vi "ClearAll.vi"(8 "error in":errorcluster) -> (0 "error out":errorcluster)   [LabVIEW 2016]
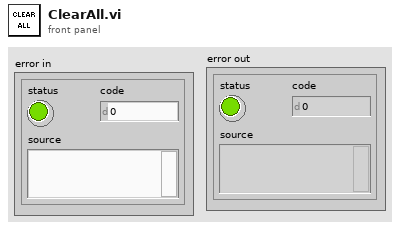
[diagram p1: front panel]
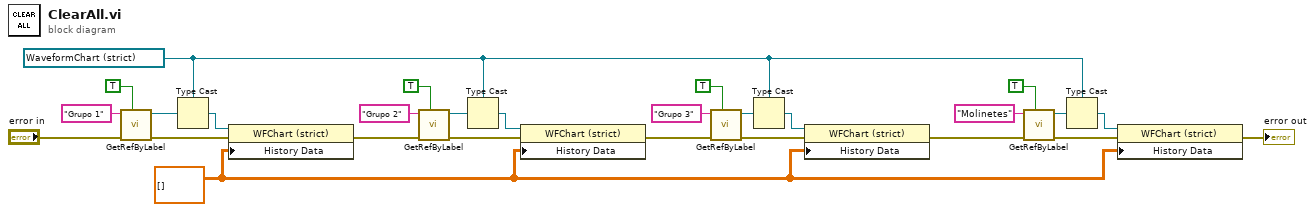
[diagram p0: block diagram]
diagram:
  w4 = dbl[][] [] ("History Data")
  w2 = refnum<vi> refnum ("Grupo 1")
  n1 = call "GetRefByLabel.vi"("InsideTab"=TRUE, "error in"="error in", "Label"="Grupo 1") -> ("error out"=w19:errorcluster, "Ctl Refnum"=w21:refnum<vi>)  [unwired: 6 in, 1 out]
  n2 = Type Cast(type=w2, x=w21) -> (*(type *) &x=w18:refnum<vi>)
  n3 = property class="WFChart (strict)"(reference=w18, error in=w19, "History Data"=w4) -> (error out=w17:errorcluster)  [unwired: 1 out]
  n4 = call "GetRefByLabel.vi"("InsideTab"=TRUE, "error in"=w17, "Label"="Grupo 2") -> ("error out"=w15:errorcluster, "Ctl Refnum"=w16:refnum<vi>)  [unwired: 6 in, 1 out]
  n5 = Type Cast(type=w2, x=w16) -> (*(type *) &x=w14:refnum<vi>)
  n6 = property class="WFChart (strict)"(reference=w14, error in=w15, "History Data"=w4) -> (error out=w13:errorcluster)  [unwired: 1 out]
  n7 = call "GetRefByLabel.vi"("InsideTab"=TRUE, "error in"=w13, "Label"="Grupo 3") -> ("error out"=w11:errorcluster, "Ctl Refnum"=w12:refnum<vi>)  [unwired: 6 in, 1 out]
  n8 = Type Cast(type=w2, x=w12) -> (*(type *) &x=w10:refnum<vi>)
  n9 = property class="WFChart (strict)"(reference=w10, error in=w11, "History Data"=w4) -> (error out=w3:errorcluster)  [unwired: 1 out]
  n10 = call "GetRefByLabel.vi"("InsideTab"=TRUE, "error in"=w3, "Label"="Molinetes") -> ("error out"=w8:errorcluster, "Ctl Refnum"=w7:refnum<vi>)  [unwired: 6 in, 1 out]
  n11 = Type Cast(type=w2, x=w7) -> (*(type *) &x=w9:refnum<vi>)
  n12 = property class="WFChart (strict)"(reference=w9, error in=w8, "History Data"=w4) -> (error out=→"error out":errorcluster)  [unwired: 1 out]
